vi "New Camera Settings.vi"(8 "error in (no error)":errorcluster, 10 "Camera Settings":variant, 11 "HIJ Vision Camera App in":refnum<class "HIJ Vision Camera App.lvclass">) -> (0 "error out":errorcluster, 3 "HIJ Vision Camera App out":refnum<class "HIJ Vision Camera App.lvclass">)   [LabVIEW 2014, in "HIJ Vision Camera App.lvlib" / "HIJ Vision Camera App.lvclass"]
uses:
  HIJ Vision Camera App.lvclass
  HIJ Vision Camera App.lvclass/HIJ Vision Camera App.ctl
  HIJ Vision Application/HIJ Vision Application/HIJ Vision Application.lvclass/HIJ Vision Application.ctl
  Camera Actors/Camera Actor/Camera Actor Messages/Publish Camera Settings Msg/Publish Camera Settings Msg.lvclass/Publish Camera Settings Msg.ctl
  <vilib>/ActorFramework/Message Enqueuer/Message Enqueuer.lvclass/Message Enqueuer.ctl
  HIJ Vision Application/HIJ Vision Application/Read Display Enq.vi
  <vilib>/ActorFramework/Message Enqueuer/Enqueue.vi
  <vilib>/ActorFramework/Message Priority Queue/Priority Enqueue.vi
  <vilib>/ActorFramework/Message Enqueuer/Message Enqueuer.lvclass
  Camera Actors/Camera Actor/Camera Actor Messages/Publish Camera Settings Msg/Publish Camera Settings Msg.lvclass
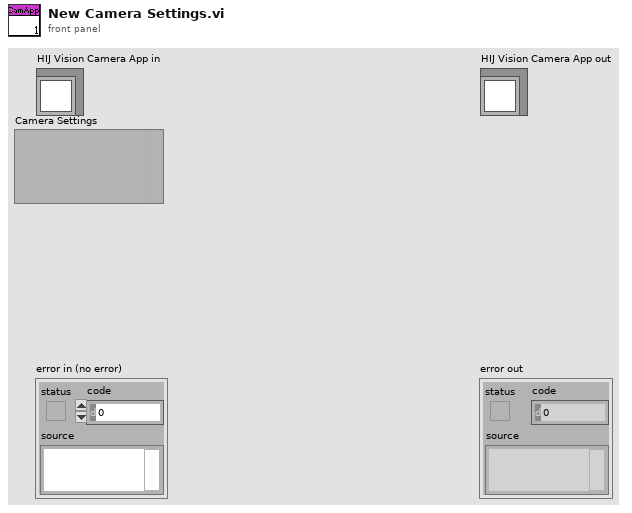
[diagram p1: front panel]
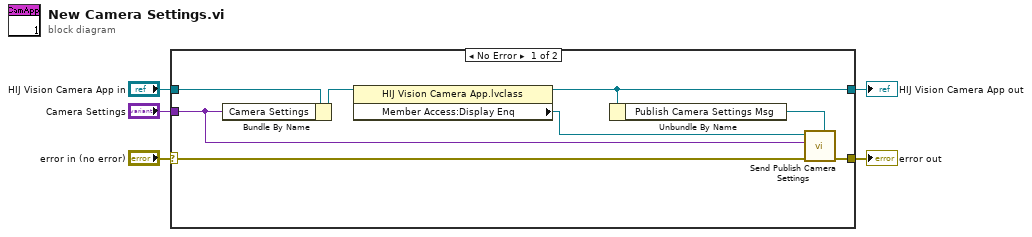
[diagram p0: block diagram]
diagram:
  n1 = case shown="No Error" "error in (no error)" {
    selector: "error in (no error)" -> [w7 w15]
    tunnel: [w6 w15] -> w4
    tunnel: [w11 w14] -> w2
    tunnel: "HIJ Vision Camera App in" -> [w13 w14]
    tunnel: "Camera Settings" -> [w8 _]
    frame No Error {
      n2 = Bundle By Name(cluster=w13, "Camera Settings"=w8) -> (w12:refnum<class "HIJ Vision Camera App.lvclass">)
      n3 = property class="HIJ Vision Camera App.lvclass"(reference=w12) -> (reference out=w11:refnum<class "HIJ Vision Camera App.lvclass">, "Member Access:Display Enq"=w10:refnum<class "Message Enqueuer.lvclass">)  [unwired: 1 in, 1 out]
      n4 = Unbundle By Name(w11) -> ("Publish Camera Settings Msg"=w9:refnum<class "Publish Camera Settings Msg.lvclass">)
      n5 = call "Send Publish Camera Settings.vi"("Message Type"=w9, "error in (no error)"=w7, "Camera Settings"=w8, "Message Enqueuer"=w10) -> ("error out"=w6:errorcluster)  [unwired: 6 in, 1 out]
    }
    frame Error {
    }
  }
  "error out" <- w4
  "HIJ Vision Camera App out" <- w2
